vi "gamb_MDC.vi"(6 "Controle sentido M2":bool, 7 "Ligar (StandBy)":bool, 8 "error in (no error)":errorcluster, 9 "Duty Cycle MCC2 : Faixa de operação  in":dbl(slide) scale=0.0..1.0, 10 "Duty Cycle MCC1 : Faixa de operação in":dbl(slide) scale=0.0..1.0, 11 "Controle sentido M1":bool) -> (2 "Duty Cycle MCC1 : Faixa de operação out":dbl, 3 "Duty Cycle MCC2 : Faixa de operação  out":dbl)   [LabVIEW 2017]
uses:
  <vilib>/myRIO/Instrument Drivers/Onboard IO/PWM/typedefs/PWM Reference.ctl
  <vilib>/myRIO/Common/Instrument Driver Framework/Utilities/typedefs/myRIO Generic Hardware Reference.ctl
  <vilib>/myRIO/Common/Instrument Driver Framework/Utilities/typedefs/Hardware Version Enum.ctl
  <vilib>/myRIO/Common/Instrument Driver Framework/Utilities/typedefs/myRIO v1.0 Reference.ctl
  <vilib>/myRIO/Common/Instrument Driver Framework/Utilities/typedefs/Generic FPGA Reference.ctl
  <vilib>/myRIO/Common/Instrument Driver Framework/myRIO v1.0/PWM/typedefs/PWM Channels Enum.ctl
  <vilib>/myRIO/Instrument Drivers/Onboard IO/PWM/typedefs/PWM Configuration.ctl
  <vilib>/userdefined/High Color/nirio_resource_hc.ctl
  <vilib>/myRIO/Instrument Drivers/Onboard IO/DIO/typedefs/DIO Reference.ctl
  <vilib>/myRIO/Common/Instrument Driver Framework/myRIO v1.0/DIO/typedefs/DIO Channels List.ctl
  <vilib>/myRIO/Common/Instrument Driver Framework/myRIO v1.0/DIO/typedefs/DIO Channels Enum.ctl
  <vilib>/myRIO/Common/Instrument Driver Framework/Utilities/vis/Is FPGA Ref Available.vi
  <vilib>/myRIO/Common/Instrument Driver Framework/myRIO v1.0/DIO/vis/myRIO v1.1 Open DIO.vi
  <vilib>/myRIO/Instrument Drivers/Onboard IO/DIO/vis/Write.vi
  <vilib>/myRIO/Common/Instrument Driver Framework/myRIO v1.0/PWM/vis/myRIO v1.1 Open PWM.vi
  <vilib>/myRIO/Instrument Drivers/Onboard IO/PWM/vis/Set Duty Cycle and Frequency.vi
  <vilib>/myRIO/Common/Instrument Driver Framework/Utilities/vis/Validate Channels.vi
  <vilib>/myRIO/Common/Instrument Driver Framework/myRIO v1.0/DIO/vis/myRIO v1.0 Reserve DIO.vi
  <vilib>/myRIO/Common/Instrument Driver Framework/myRIO v1.0/PWM/vis/myRIO v1.0 Reserve PWM.vi
  <vilib>/myRIO/Common/Instrument Driver Framework/myRIO v1.0/Resource Manager/vis/myRIO v1.0 Reserve Channel List.vi
  <vilib>/myRIO/Common/Instrument Driver Framework/myRIO v1.0/DIO/vis/myRIO v1.0 Build MUX Configuration DIO.vi
  <vilib>/myRIO/Common/Instrument Driver Framework/myRIO v1.0/PWM/vis/myRIO v1.0 Build MUX Configuration PWM.vi
  <vilib>/myRIO/Common/Instrument Driver Framework/myRIO v1.0/Resource Manager/vis/myRIO v1.0 Reserve Channel.vi
  <vilib>/myRIO/Common/Instrument Driver Framework/myRIO v1.0/Resource Manager/vis/myRIO v1.0 Unreserve Channel.vi
  <vilib>/myRIO/Common/Instrument Driver Framework/myRIO v1.0/Resource Manager/vis/myRIO v1.0 Create Configuration List.vi
  <vilib>/myRIO/Common/Instrument Driver Framework/myRIO v1.0/Resource Manager/vis/myRIO v1.0 Build Mutex Name.vi
  <vilib>/Utility/VariantDataType/GetNumericInfo.vi
  <vilib>/Utility/error.llb/Error Cluster From Error Code.vi
  <vilib>/myRIO/Common/Instrument Driver Framework/myRIO v1.0/myRIO v1.1 Open.vi
  <vilib>/myRIO/Common/Instrument Driver Framework/Utilities/vis/IO Manager.vi
  <vilib>/myRIO/Common/Instrument Driver Framework/Utilities/vis/Configuration Manager.vi
  <vilib>/myRIO/Common/Instrument Driver Framework/myRIO v1.0/Resource Manager/vis/myRIO v1.0 Configure IO.vi
  <vilib>/myRIO/Common/Instrument Driver Framework/myRIO v1.0/myRIO v1.0 Close.vi
  <vilib>/myRIO/Common/Instrument Driver Framework/myRIO v1.0/DIO/vis/myRIO v1.0 Write DIO.vi
  <vilib>/myRIO/Common/Instrument Driver Framework/myRIO v1.0/PWM/vis/myRIO v1.0 Write PWM.vi
  <vilib>/myRIO/Express VI/Onboard Devices/LED/LED Express VI.xnode
  <vilib>/myRIO/Instrument Drivers/Onboard IO/DIO/vis/myRIO DIO Open.xnode
  <vilib>/myRIO/Express VI/Onboard IO/PWM/PWM Express VI.xnode
  <vilib>/myRIO/Instrument Drivers/Onboard IO/PWM/vis/myRIO PWM Open.xnode
  <vilib>/myRIO/Express VI/Onboard IO/DO/DO Express VI.xnode
  <vilib>/myRIO/Instrument Drivers/Onboard IO/DIO/DIO.lvlib
  <vilib>/myRIO/Instrument Drivers/Onboard IO/PWM/PWM.lvlib
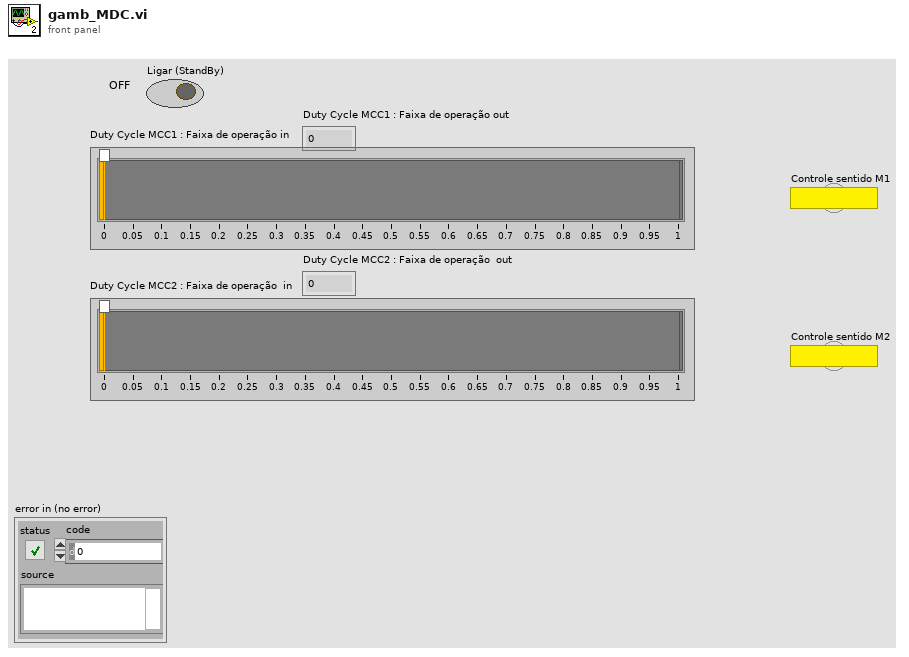
[diagram p1: front panel]
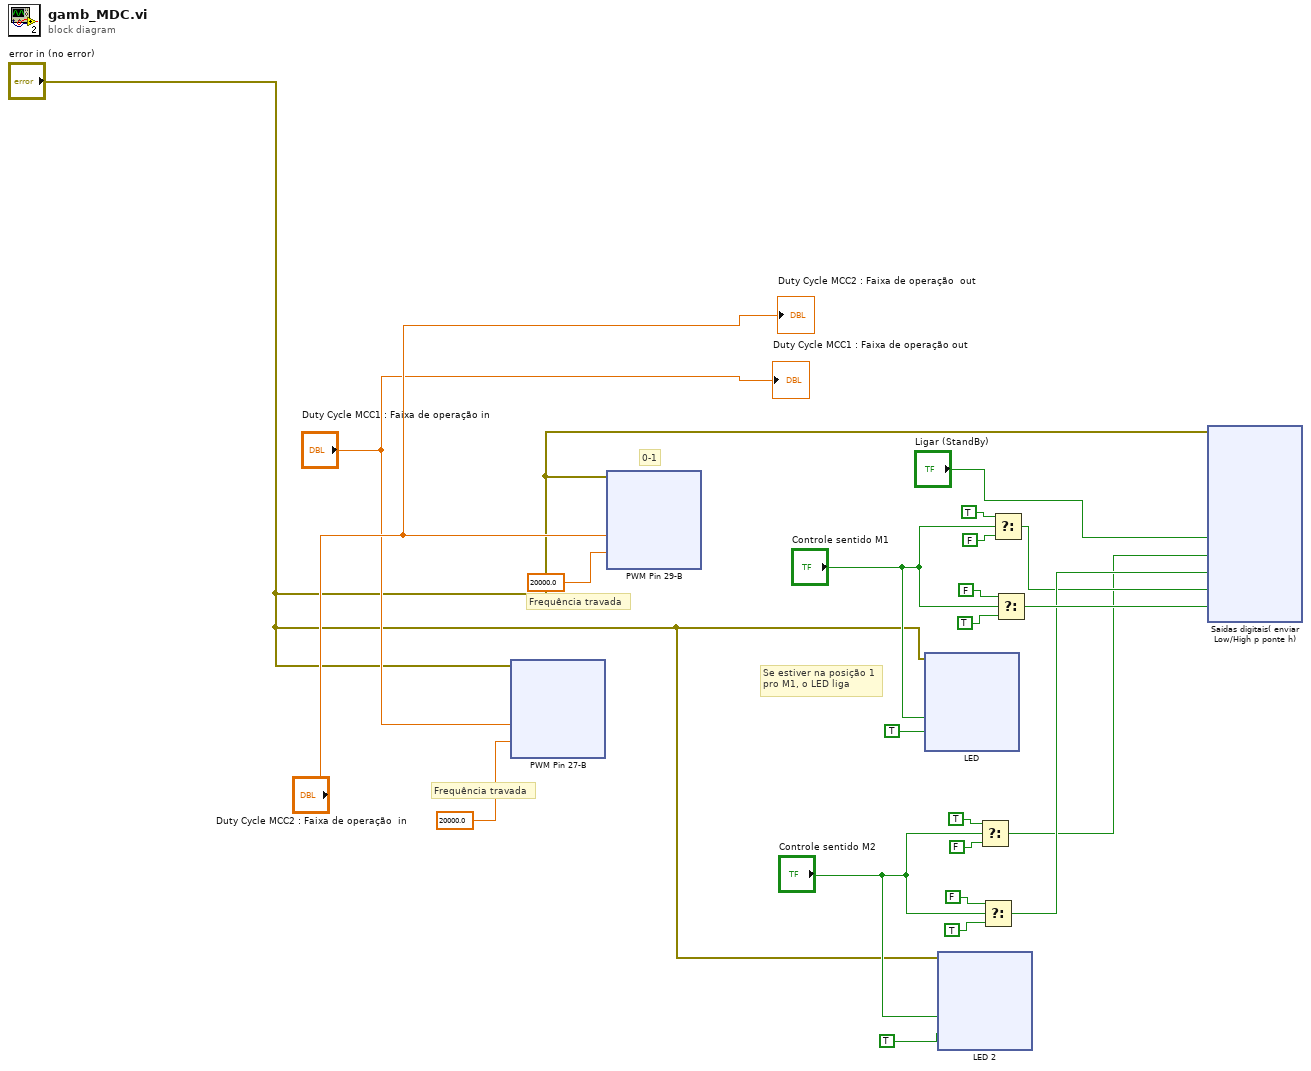
[diagram p0: block diagram]
diagram:
  # "Frequência travada"
  # "Se estiver na posição 1\npro M1, o LED liga"
  # "Frequência travada"
  # "0-1"
  n1 = xnode "PWM Pin 27-B"("Duty Cycle"="Duty Cycle MCC1 : Faixa de operação in", "Frequency [Hz]"=20000.0, "error in (no error)"="error in (no error)") -> ()  [unwired: 1 out]
  n2 = xnode "PWM Pin 29-B"("Duty Cycle"="Duty Cycle MCC2 : Faixa de operação  in", "Frequency [Hz]"=20000.0, "error in (no error)"="error in (no error)") -> ()  [unwired: 1 out]
  n3 = xnode "LED"("LED0"="Controle sentido M1", "LED1"=TRUE, "error in (no error)"="error in (no error)") -> ()  [unwired: 1 out]
  n4 = xnode "LED 2"("LED2"="Controle sentido M2", "LED3"=TRUE ("LED1"), "error in (no error)"="error in (no error)") -> ()  [unwired: 1 out]
  n5 = Select(t=TRUE ("Controle sentido"), s="Controle sentido M2", f=FALSE ("Controle sentido")) -> (s? t:f=w17:bool)
  n6 = Select(t=FALSE ("Controle sentido"), s="Controle sentido M2", f=TRUE ("Controle sentido")) -> (s? t:f=w19:bool)
  n7 = Select(t=TRUE ("Controle sentido"), s="Controle sentido M1", f=FALSE ("Controle sentido")) -> (s? t:f=w18:bool)
  n8 = Select(t=FALSE ("Controle sentido"), s="Controle sentido M1", f=TRUE ("Controle sentido")) -> (s? t:f=w20:bool)
  n9 = xnode "Saídas digitais( enviar Low/High p ponte h)"("Standby (B/DIO7 (Pin 25))"="Ligar (StandBy)", "M2 A (B/DIO15 (Pin 34))"=w17, "M2 B (B/DIO14 (Pin 32))"=w19, "M1 A (B/DIO13 (Pin 26))"=w18, "M1 B (B/DIO12 (Pin 22))"=w20, "error in (no error)"="error in (no error)") -> ()  [unwired: 1 out]
  "Duty Cycle MCC2 : Faixa de operação  out" <- "Duty Cycle MCC2 : Faixa de operação  in"
  "Duty Cycle MCC1 : Faixa de operação out" <- "Duty Cycle MCC1 : Faixa de operação in"
